vi "AutoRun.vi"(11 "AllControls In":T2) -> ()   [LabVIEW 2017]
uses:
  Ctrls/AllControls.ctl
  Ctrls/CSV_Data.ctl
  Ctrls/NFC.bat
  <vilib>/Utility/miscctls.llb/LVRowAndColumnTypeDef.ctl
  Ctrls/PathChoose.ctl
  ComVIS/Files/Ini/WriteIniFiles_ByVarient.vi
  <vilib>/Utility/file.llb/Write Delimited Spreadsheet (string).vi
  <vilib>/regexp/Match Regular Expression.xnode
panel:
  in  "Data in 2":T1
  in  "Data in":T1
types:
  T1 = typedef "CSV_Data.ctl" = cluster{"Version":cluster{"SC_Version":string, "VP_Version":string}, "SN":string, "Table":string[][], "Count":cluster{"Total":i32, "OK":i32, "NG":i32, "Yield":dbl}, "Start Time":timestamp, "daemon reference":refnum<k5>, "CT":dbl, "Config":string[][], "OK/NG":bool, "Station ID":string, "MES DDM SN":string, "MES PCBA SN":string, "Retest":string, "Lux":string, "VOT":cluster{"Initial brightness":string, "Mean uniformity":string, "Uniformity_Deviation":string, "Adjusted brightness":string, "Mean_Adjusted":string, "Deviation_Adjusted":string, "Reflection":string, "Result":bool}, "SKU":string, "Plate_Diameter":string, "Alarm":string}
  T2 = typedef "AllControls.ctl" = cluster{"MainVI":refnum<vi>, "AlarmInfo":refnum<vi>, "Log":refnum<vi>, "Current CT":refnum<vi>, "ProductID":refnum<vi>, "Device state":refnum<vi>, "MES":refnum<vi>, "mode":refnum<vi>, "TestInfo":refnum<vi>, "SubPnl":refnum<vi>, "Table":refnum<vi>, "MES bool":refnum<vi>, "TestMode":refnum<vi>, "Recipe":refnum<vi>, "Fail resume":refnum<vi>, "LogIn":refnum<vi>, "Start":refnum<vi>, "Maintenance":refnum<vi>, "Stop":refnum<vi>, "Exit":refnum<vi>}
  T3 = typedef "NFC.bat" = cluster{"getVersion":string, "Start Test mode":string, "Start camera test mode":string, "get one RAW Image":string, "Stop camera test mode":string, "Stop Test Mode":string, "Get image reflection":string, "Get image uniformity andFlash LED brightness":string, "Disable flash LED":string, "Enable flash LED":string, "Software Reset":string, "Tune Flash LED brightness":string, "Start Camera calibration":string, "Verify OBC Setting":string}
  T4 = typedef "amc_Message Queue.ctl" = refnum<queue>
  T5 = typedef "TesterInfo.ctl" = cluster{"Station Name":string, "Station Code":string, "ES NO.":string, "Tester ID":string, "PassMark Revision":string, "Rig ID":string, "682_Tool_Repeat":string, "Project Name":string, "FFTesterPath":path, "Enable_User":bool, "Mode":enum16{"682"}, "Fail_resume_mode":bool}
  T6 = cluster{"Total":i32, "OK":i32, "NG":i32, "Yield":dbl}
  T7 = typedef "LVRowAndColumnTypeDef.ctl" = cluster{"Row":i32, "Column":i32}
  T8 = enum8{"Enabled", "Disabled", "Disabled and Grayed Out"}
  T9 = typedef "PathChoose.ctl" = enum16{"OperatorLog", "AutoRunLog", "AlmLog", "TestData", "AllTestData", "backup_nvm", "backup_before_flashing"}
  T10 = typedef "HD Config.ctl" = cluster{" PC":cluster{"PC Address":u8[], "PC Port":i32}, "FCO":cluster{"COM":refnum<visa-resource-name>, "Baudrate":u32}, "DC Power ":cluster{"COM":refnum<visa-resource-name>, "Baudrate":u32}, "PW3336":cluster{"COM":refnum<visa-resource-name>, "Baudrate":u32}, "Lefoo":cluster{"COM":refnum<visa-resource-name>, "Baudrate":u32}, "Tempt&Hum":cluster{"COM":refnum<visa-resource-name>, "Baudrate":u32}, "DIPC":cluster{"COM":refnum<visa-resource-name>}, "Daemon":cluster{"IP Address":string, "Port":u16, "Retry":u16}, "NFC_Cmd":cluster{"COM":refnum<visa-resource-name>, "Baudrate":u32}, "Fail_resume_mode":bool, "GRR":bool, "NFC _Serial":cluster{"COM":refnum<visa-resource-name>, "Baudrate":u32}}
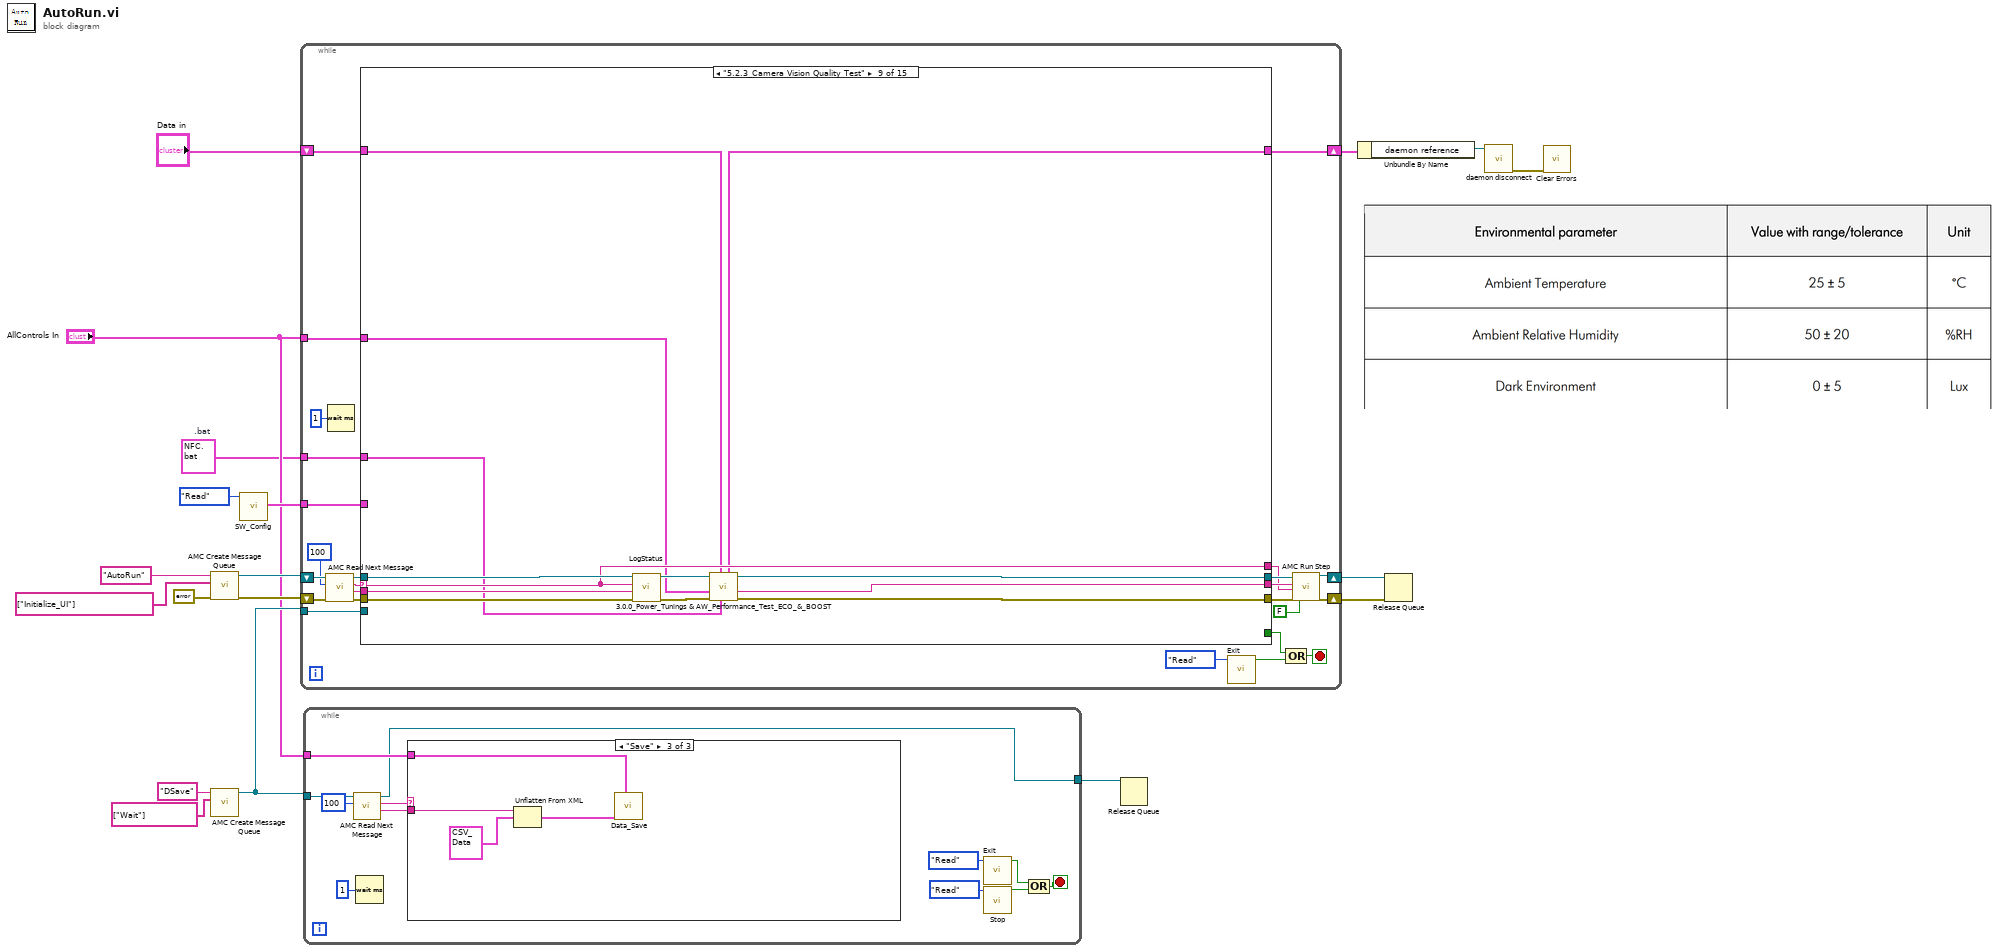
[diagram p0: block diagram]
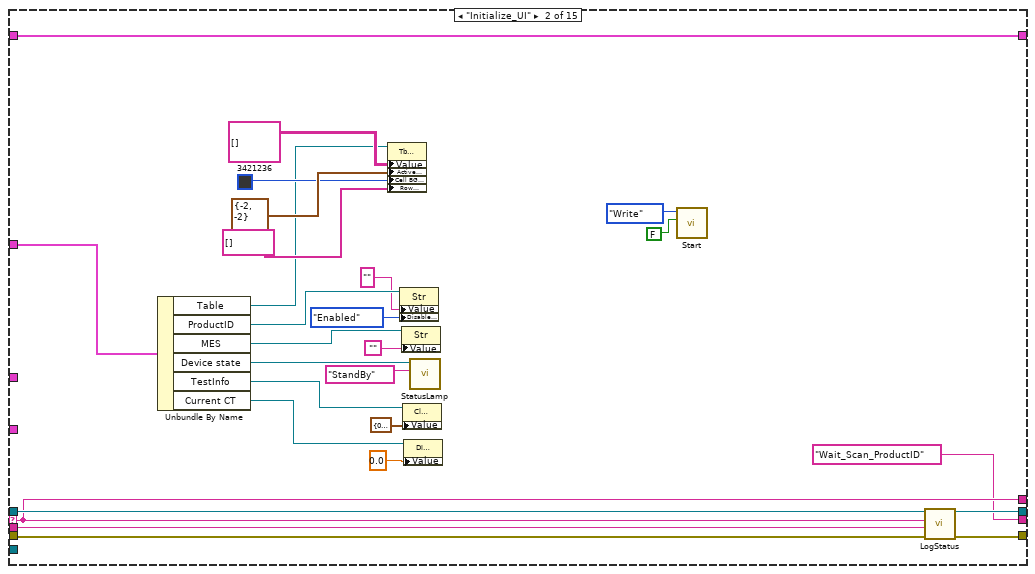
[diagram p5: hidden frame]
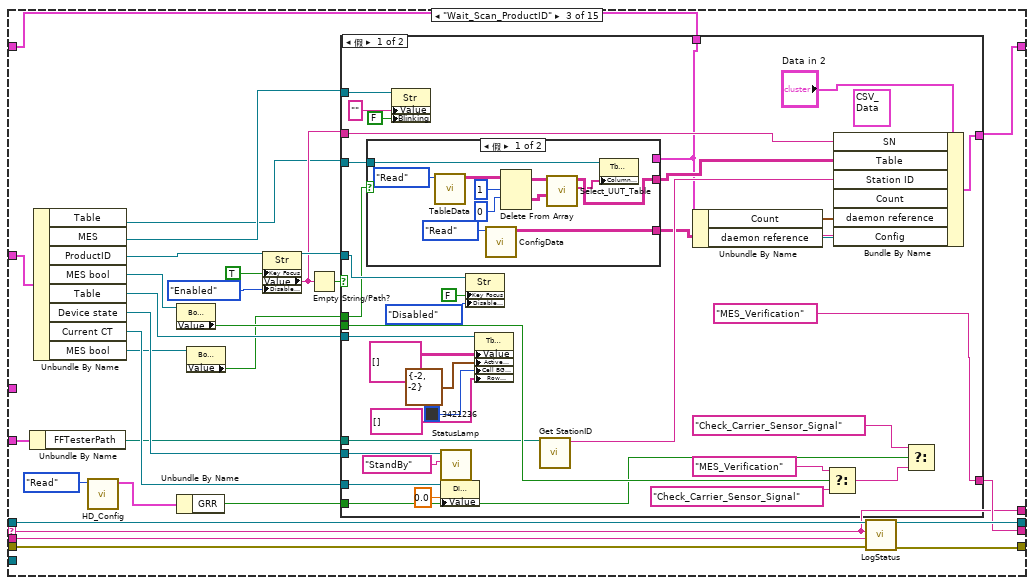
[diagram p6: hidden frame]
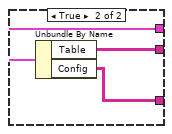
[diagram p7: hidden frame]
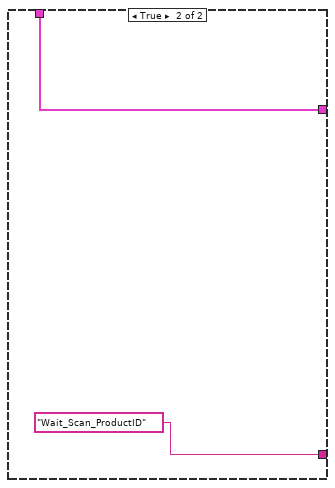
[diagram p8: hidden frame]
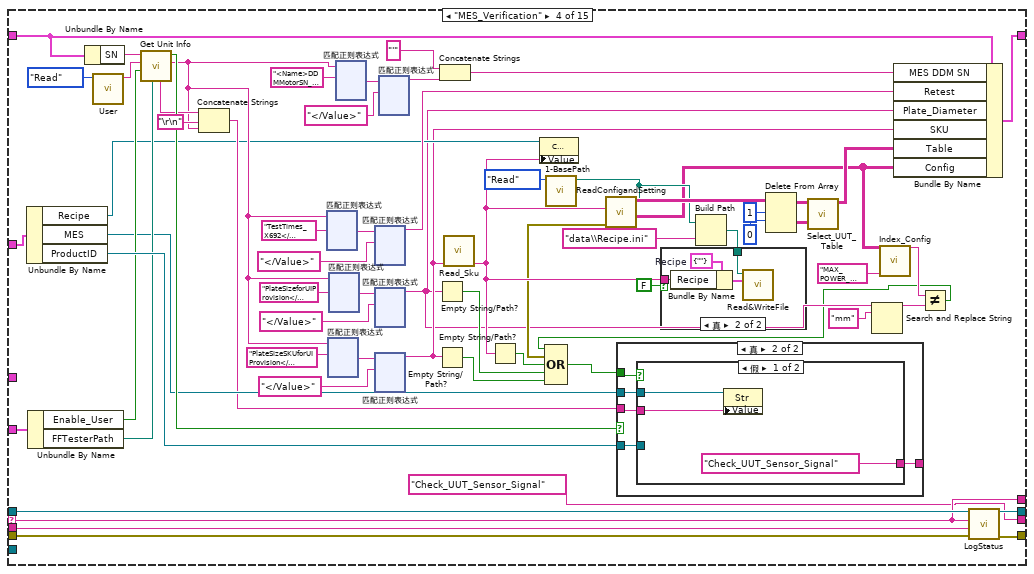
[diagram p9: hidden frame]
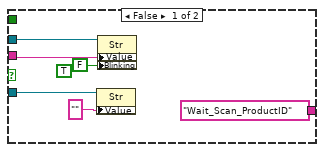
[diagram p11: hidden frame]
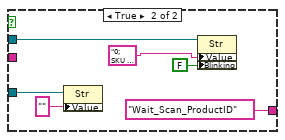
[diagram p12: hidden frame]
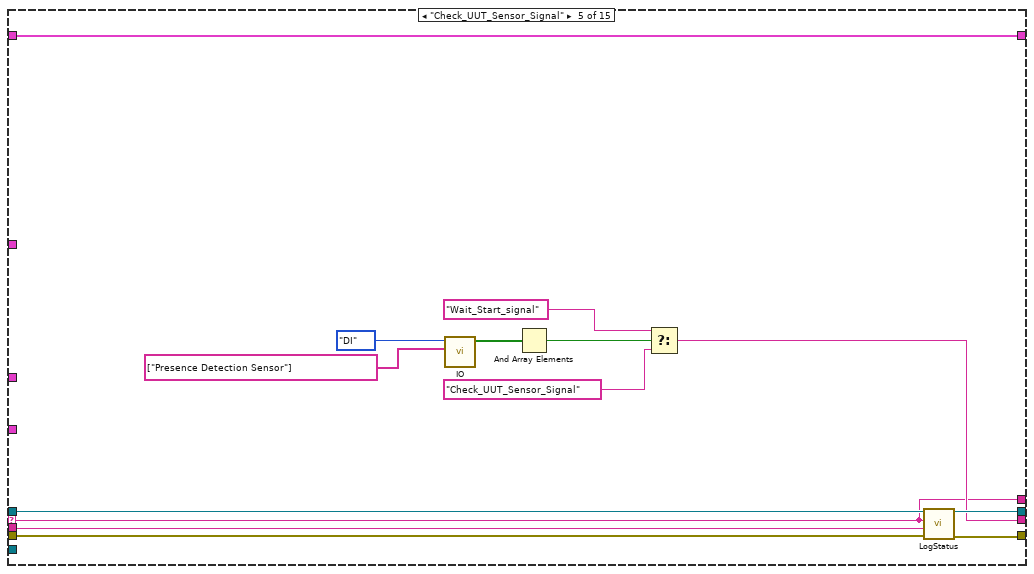
[diagram p13: hidden frame]
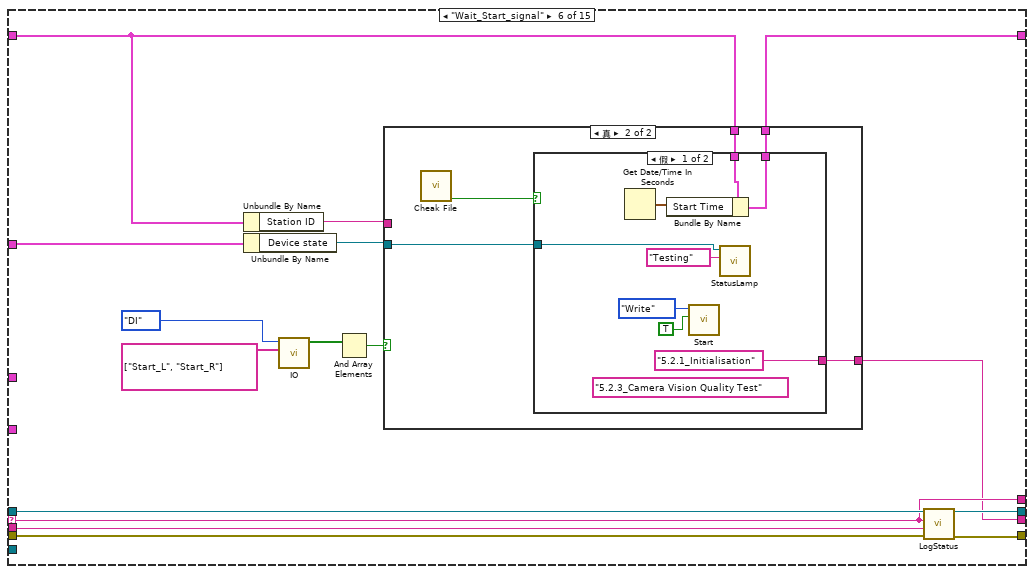
[diagram p14: hidden frame]
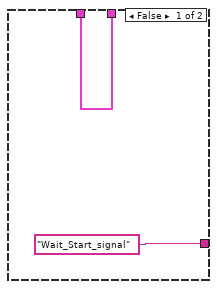
[diagram p15: hidden frame]
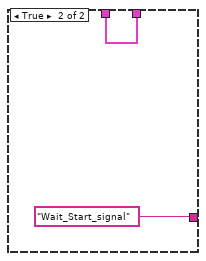
[diagram p16: hidden frame]
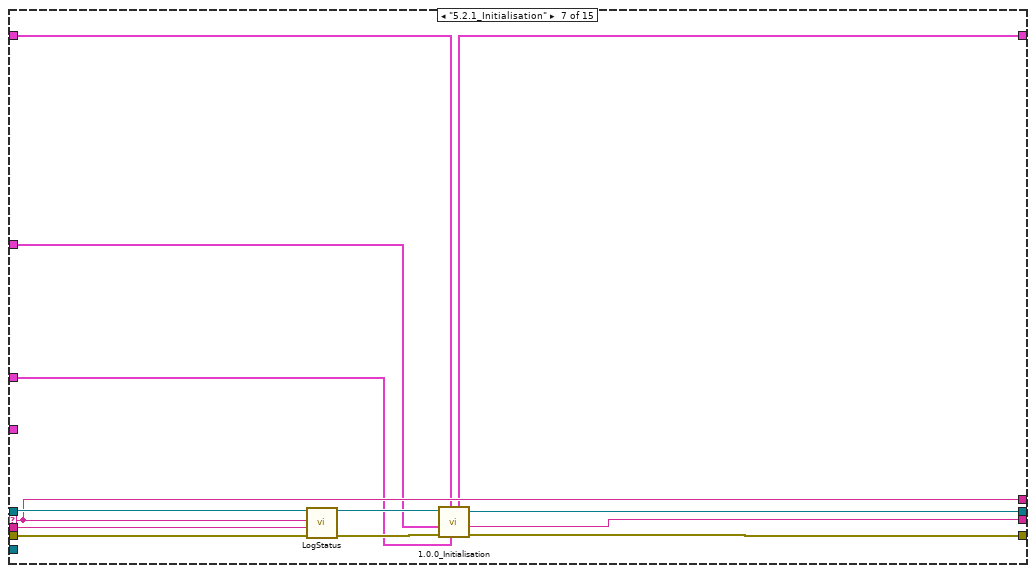
[diagram p17: hidden frame]
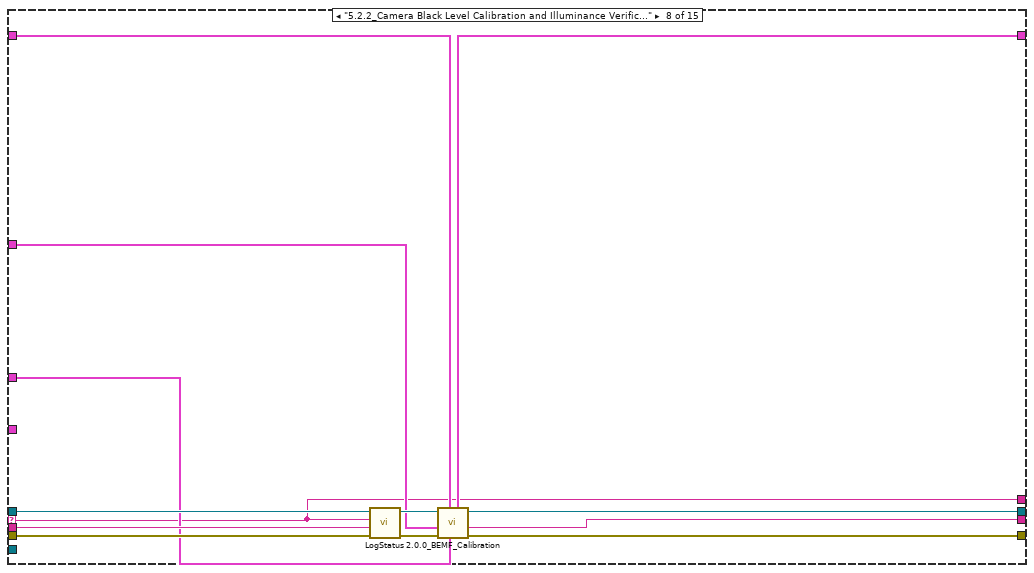
[diagram p18: hidden frame]
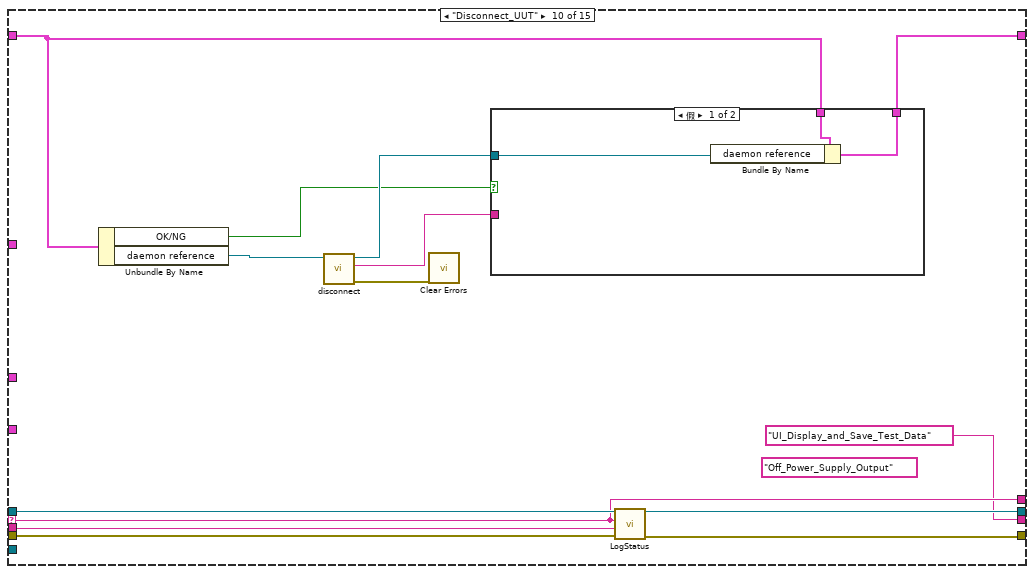
[diagram p19: hidden frame]
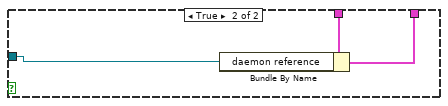
[diagram p20: hidden frame]
diagram:
  w1 = T3 {"getVersion"="Getting Software Version.bat", "Start Test mode"="Start Test Mode.bat", "Start camera test mode"="Start camera test mode.bat", "get one RAW Image"="Get one image.bat", "Stop camera test mode"="Stop camera test mode.bat", "Stop Test Mode"="Stop Test Mode.bat", "Get image reflection"="Get image reflection.bat", "Get image uniformity andFlash LED brightness"="Get image uniformity andFlash LED brightness.bat", "Disable flash LED"="Disable flash LED.bat", "Enable flash LED"="Enable flash LED.bat", "Software Reset"="Software Reset.bat", "Tune Flash LED brightness"="Tune Flash LED brightness.bat", "Start Camera calibration"="Start Camera calibration.bat", "Verify OBC Setting"="Verify OBC Setting.bat"}  # .bat
  n1 = call "AMC Create Message Queue.vi"("error in (no error)"=errorcluster {"status"=FALSE, "code"=0, "source"=""}, "Initial Message Names"=string[] ["Initialize_UI"] ("Initial Message Values"), "Message Queue Name"="AutoRun" ("Message queue name (unnamed)")) -> ("error out"=w17:errorcluster, "Message Queue out"=w18:T4)  [unwired: 2 in, 5 out]
  n2 = call "AMC Create Message Queue.vi"("Initial Message Names"=string[] ["Wait"], "Message Queue Name"="DSave") -> ("Message Queue out"=w13:T4)  [unwired: 3 in, 6 out]
  n3 = call "SW_Config.vi"("Step"=enum16{"Initial", "Write", "Read"}."Read") -> ("SW Config out"=w9:T5)  [unwired: 9 in, 1 out]
  n4 = while {
    tunnel: "AllControls In" -> [w30]
    shift-right: [w39] -> w6
    shift-left: w18 -> [w44]
    shift-right: [w40] -> w5
    shift-left: w17 -> [w43]
    tunnel: w13 -> [w35]
    tunnel: w9 -> [w23]
    shift-right: [w22] -> w8
    shift-left: "Data in" -> [w21]
    tunnel: w1 -> [w20]
    stop <- w38 stop-if-true
    n5 = call "AMC Read Next Message.vi"("error in (no error)"=w43, "timeout (1ms)"=100 ("Timeout"), "Message Queue in"=w44) -> ("error out"=w31:errorcluster, "Message Value"=w24:string, "Message Name"=w34:string, "Message Queue out"=w33:T4)  [unwired: 1 in, 4 out]
    n6 = Wait (ms)(milliseconds to wait=u32 1) -> ()  [unwired: 1 out]
    n7 = case shown="\"5.2.3_Camera Vision Quality Test\"" w34 {
      selector: w34 -> [_ w49 w90 w210 w1158 w1175 w1204 w1210 w1228 w1243 w1295 w1317 w1355 w1365 w1423]
      tunnel: w35 -> [_ _ _ _ _ _ _ _ _ _ w1299 _ _ _ _]
      tunnel: w33 -> [w47 w73 w102 w216 w1165 w1180 w1207 w1219 w1231 w1246 w1300 w1322 w1358 w1388 w1425]
      tunnel: [w47 w73 w102 w216 w1165 w1180 w1206 w1218 w1230 w1246 w1300 w1322 w1358 w1388 w1425] -> w32
      tunnel: w31 -> [w46 w53 w101 w215 w1164 w1179 w1209 w1221 w1233 w1245 w1297 w1321 w1357 w1387 w1421]
      tunnel: [w46 w69 w100 w214 w1163 w1178 w1205 w1217 w1229 w1244 w1296 w1320 w1356 w1386 w1422] -> w27
      tunnel: w30 -> [_ w71 w96 w212 _ w1171 w1202 w1214 w1225 _ w1286 w1302 w1346 w1376 _]
      tunnel: [_ _ _ _ _ _ _ _ _ _ _ _ _ _ TRUE] -> w29
      tunnel: [_ "Wait_Scan_ProductID" w94 "Check_UUT_Sensor_Signal" w1159 w1169 w1199 w1215 w1226 "UI_Display_and_Save_Test_Data" w1253 "Wait_Scan_ProductID" w1347 w1375 _] -> w26
      tunnel: [_ w49 w90 w210 w1158 w1175 w1204 w1210 w1228 w1243 w1295 w1317 w1355 w1365 _] -> w25
      tunnel: w24 -> [_ w63 w92 w211 w1157 w1174 w1208 w1220 w1232 w1242 w1294 w1318 w1354 w1364 _]
      tunnel: w23 -> [_ _ w83 w205 _ _ _ _ _ _ _ w1304 _ _ _]
      tunnel: [w45 w50 w81 w201 w1153 w1166 w1201 w1213 w1223 w1239 w1260 w1301 w1331 w1369 w1420] -> w22
      tunnel: w21 -> [w45 w50 w80 w202 w1153 w1167 w1200 w1212 w1224 w1238 w1259 w1301 w1331 w1370 w1420]
      tunnel: w20 -> [_ _ _ _ _ _ w1198 w1211 w1222 _ _ _ _ _ _]
      frame "Empty", Default {
      }
      frame "Initialize_UI" {
        n8 = Unbundle By Name(w71) -> ("Table"=w58:refnum<vi>, "ProductID"=w66:refnum<vi>, "MES"=w72:refnum<vi>, "Device state"=w68:refnum<vi>, "TestInfo"=w57:refnum<vi>, "Current CT"=w55:refnum<vi>)
        n9 = property class="Tbl (strict)"(reference=w58, "Value"=string[][] [] ("值"), "Active Cell"=T7 {"Row"=-2, "Column"=-2} ("活动单元格:活动单元格"), "Cell BG Color"=u32 3421236, "Row Headers[]"=string[] [] ("Row Header Strings[]")) -> ()  [unwired: 1 in, 2 out]
        n10 = property class="Str"(reference=w66, "Value"="" ("值"), "DisabledEnum"=T8."Enabled" ("Disabled")) -> ()  [unwired: 1 in, 2 out]
        n11 = property class="Str"(reference=w72, "Value"="") -> ()  [unwired: 1 in, 2 out]
        n12 = property class="Clust (strict)"(reference=w57, "Value"=T6 {"Total"=0, "OK"=0, "NG"=0, "Yield"=0.0}) -> ()  [unwired: 1 in, 2 out]
        n13 = property class="DigNum (strict)"(reference=w55, "Value"=0.0) -> ()  [unwired: 1 in, 2 out]
        n14 = call "StatusLamp.vi"("State"="StandBy", "Boolean输入"=w68) -> ()  [unwired: 9 in, 1 out]
        n15 = call "Start.vi"("Start In"=FALSE, "Step"=enum16{"Initial", "Write", "Read"}."Write") -> ()  [unwired: 8 in, 2 out]
        n16 = call "LogStatus.vi"("error in (no error)"=w53, "last message"=w63, "message"=w49) -> ("error  out"=w69:errorcluster)  [unwired: 8 in]
      }
      frame "Wait_Scan_ProductID" {
        n17 = Unbundle By Name(w83) -> ("FFTesterPath"=w82:path)
        n18 = Unbundle By Name(w96) -> ("Table"=w74:refnum<vi>, "MES"=w87:refnum<vi>, "ProductID"=w99:refnum<vi>, "MES bool"=w89:refnum<vi>, "Table"=w86:refnum<vi>, "Device state"=w85:refnum<vi>, "Current CT"=w84:refnum<vi>, "MES bool"=w76:refnum<vi>)
        n19 = call "HD_Config.vi"("Step"=enum16{"Initial", "Write", "Read"}."Read") -> ("HD Config out"=w78:T10)  [unwired: 9 in, 1 out]
        n20 = property class="Bool (strict)"(reference=w89) -> ("Value"=w88:bool)  [unwired: 1 in, 2 out]
        n21 = Unbundle By Name(w78) -> ("GRR"=w77:bool)
        n22 = property class="Bool (严格)"(reference=w76) -> ("Value"=w75:bool)  [unwired: 1 in, 2 out]
        n23 = property class="Str"(reference=w99, "Key Focus"=TRUE, "DisabledEnum"=T8."Enabled" ("Disabled")) -> (reference out=w93:refnum<vi>, "Value"=w91:string)  [unwired: 1 in, 1 out]
        n24 = Empty String/Path?(string/path=w91) -> (empty?=w95:bool)
        n25 = case shown="假" w95 {
          tunnel: ["MES_Verification" "Wait_Scan_ProductID"] -> w94
          tunnel: w93 -> [w134 _]
          tunnel: w91 -> [w117 _]
          tunnel: w88 -> [w131 _]
          tunnel: w87 -> [w130 _]
          tunnel: w86 -> [w124 _]
          tunnel: w85 -> [w122 _]
          tunnel: w84 -> [w121 _]
          tunnel: w82 -> [w119 _]
          tunnel: [w118 w151] -> w81
          tunnel: w80 -> [w105 w151]
          tunnel: w77 -> [w113 _]
          tunnel: w75 -> [w108 _]
          tunnel: w74 -> [w106 _]
          frame False {
            (unwired) T1 {"Version"={"SC_Version"="", "VP_Version"=""}, "SN"="", "Table"=[], "Count"={"Total"=0, "OK"=0, "NG"=0, "Yield"=0.0}, "Start Time"=timestamp(0 s since 1904-01-01), "daemon reference"=refnum, "CT"=0.0, "Config"=[], "OK/NG"=FALSE, "Station ID"="", "MES DDM SN"="", "MES PCBA SN"="", "Retest"="", "Lux"="", "VOT"={"Initial brightness"="", "Mean uniformity"="", "Uniformity_Deviation"="", "Adjusted brightness"="", "Mean_Adjusted"="", "Deviation_Adjusted"="", "Reflection"="", "Result"=FALSE}, "SKU"="", "Plate_Diameter"="", "Alarm"=""} ("Data in")
            n26 = case shown="假" w108 {
              tunnel: [w141 w149] -> w116
              tunnel: [w139 w148] -> w107
              tunnel: w106 -> [w138 _]
              tunnel: w105 -> [_ w150]
              frame False {
                n27 = call "TableData.vi"("Step"=enum16{"Initial", "Write", "Read"}."Read") -> ("Tabledata Out"=w142:string[][])  [unwired: 9 in, 1 out]
                n28 = call "ConfigData.vi"("Step"=enum16{"Initial", "Write", "Read"}."Read") -> ("Tabledata Out"=w139:string[][])  [unwired: 9 in, 1 out]
                n29 = Delete From Array(array=w142, length=1 ("长度"), index (row)=0 ("索引 (行)")) -> (deleted portion=w143:string[][], array with subset deleted=w144:string[][])  [unwired: 1 in]
                n30 = call "Select_UUT_Table.vi"("all Title"=w143, "all Table"=w144) -> ("Title"=w137:string[], "Table"=w141:string[][])  [unwired: 8 in]
                n31 = property class="Tbl (strict)"(reference=w138, "Column Headers[]"=w137) -> ()  [unwired: 1 in, 2 out]
              }
              frame True {
                n32 = Unbundle By Name(w150) -> ("Table"=w149:string[][], "Config"=w148:string[][])
              }
            }
            n33 = property class="Str"(reference=w130, "Value"="" ("值"), "Blinking"=FALSE ("闪烁")) -> ()  [unwired: 1 in, 2 out]
            n34 = call "StatusLamp.vi"("State"="StandBy", "Boolean输入"=w122) -> ()  [unwired: 9 in, 1 out]
            n35 = property class="DigNum (strict)"(reference=w121, "Value"=0.0) -> ()  [unwired: 1 in, 2 out]
            n36 = property class="Str"(reference=w134, "Key Focus"=FALSE, "DisabledEnum"=T8."Disabled" ("Disabled")) -> ()  [unwired: 1 in, 2 out]
            n37 = property class="Tbl (strict)"(reference=w124, "Value"=string[][] [] ("值"), "Active Cell"=T7 {"Row"=-2, "Column"=-2} ("活动单元格:活动单元格"), "Cell BG Color"=u32 3421236, "Row Headers[]"=string[] [] ("Row Header Strings[]")) -> ()  [unwired: 1 in, 2 out]
            n38 = call "Get StationID.vi"("路径"=w119) -> ("Station ID"=w115:string)  [unwired: 10 in]
            n39 = Unbundle By Name(w105) -> ("Count"=w111:T6, "daemon reference"=w110:refnum<k5>)
            n40 = Select(t="MES_Verification", s=w131, f="Check_Carrier_Sensor_Signal") -> (s? t:f=w114:string)
            n41 = Bundle By Name(cluster="Data in 2", "SN"=w117, "Table"=w116, "Station ID"=w115, "Count"=w111, "daemon reference"=w110, "Config"=w107) -> (w118:T1)
            n42 = Select(t="Check_Carrier_Sensor_Signal", s=w113, f=w114) -> ()  [unwired: 1 out]
          }
          frame True {
          }
        }
        n43 = call "LogStatus.vi"("error in (no error)"=w101, "last message"=w92, "message"=w90) -> ("error  out"=w100:errorcluster)  [unwired: 8 in]
      }
      frame "MES_Verification" {
        n44 = Unbundle By Name(w212) -> ("Recipe"=w167:refnum<vi>, "MES"=w188:refnum<vi>, "ProductID"=w208:refnum<vi>)
        n45 = Unbundle By Name(w205) -> ("Enable_User"=w204:bool, "FFTesterPath"=w203:path)
        n46 = Unbundle By Name(w202) -> ("SN"=w213:string)
        n47 = call "User.vi"("Step"=enum16{"Initial", "Write", "Read"}."Read") -> ("User out"=w206:string)  [unwired: 9 in, 1 out]
        n48 = call "Get Unit Info.vi"("路径"=w203, "Enable_User"=w204, "UserID"=w206, "Serial Number"=w213) -> ("strUnitInfo"=w180:string, "Operation Success"=w209:bool, "结果字符串"=w194:string)  [unwired: 2 in, 3 out]
        n49 = Concatenate Strings(w194, "\r\n", w180) -> (w187:string)
        n50 = xnode "匹配正则表达式"("输入字符串"=w180, "正则表达式"="TestTimes_X692</Name><Value>") -> ("匹配之后"=w192:string)  [unwired: 4 in, 4 out]
        n51 = xnode "匹配正则表达式"("输入字符串"=w180, "正则表达式"="PlateSizeSKUforUIProvision</Name><Value>") -> ("匹配之后"=w183:string)  [unwired: 4 in, 4 out]
        n52 = xnode "匹配正则表达式"("输入字符串"=w180, "正则表达式"="PlateSizeforUIProvision</Name><Value>") -> ("匹配之后"=w184:string)  [unwired: 4 in, 4 out]
        n53 = xnode "匹配正则表达式"("输入字符串"=w180, "正则表达式"="<Name>DDMMotorSN_X692</Name><Value>") -> ("匹配之后"=w198:string)  [unwired: 4 in, 4 out]
        n54 = xnode "匹配正则表达式"("输入字符串"=w192, "正则表达式"="</Value>") -> ("匹配之前"=w189:string)  [unwired: 4 in, 4 out]
        n55 = xnode "匹配正则表达式"("输入字符串"=w184, "正则表达式"="</Value>") -> ("匹配之前"=w156:string)  [unwired: 4 in, 4 out]
        n56 = xnode "匹配正则表达式"("输入字符串"=w183, "正则表达式"="</Value>") -> ("匹配之前"=w165:string)  [unwired: 4 in, 4 out]
        n57 = xnode "匹配正则表达式"("输入字符串"=w198, "正则表达式"="</Value>") -> ("匹配之前"=w197:string)  [unwired: 4 in, 4 out]
        n58 = Empty String/Path?(string/path=w156) -> (empty?=w179:bool)
        n59 = Empty String/Path?(string/path=w165) -> (empty?=w178:bool)
        n60 = Concatenate Strings("'", w197) -> (w196:string)
        n61 = call "Read_Sku.vi"("SKU"=w165) -> ("Recipe"=w164:string)  [unwired: 10 in]
        n62 = Empty String/Path?(string/path=w164) -> (empty?=w163:bool)
        n63 = property class="CmbBox"(reference=w167, "Value"=w164) -> ()  [unwired: 1 in, 2 out]
        n64 = call "1-BasePath.vi"("Step"=enum16{"Initial", "Write", "Read"}."Read") -> ("Path Out"=w173:path)  [unwired: 9 in, 1 out]
        n65 = call "ReadConfigandSetting.vi"("Recipe"=w164, "Path Out"=w173) -> ("错误输出"=w162:errorcluster, "ConfigData"=w157:string[][], "TableData"=w176:string[][])  [unwired: 7 in]
        n66 = Build Path(base path=w173, name or relative path="data\\Recipe.ini") -> (appended path=w172:path)
        n67 = case shown="真" FALSE {
          tunnel: w172 -> [_ w219]
          tunnel: w164 -> [_ w217]
          frame False {
          }
          frame True {
            w218 = cluster{"Recipe":string} {"Recipe"=""}  # Recipe
            n68 = Bundle By Name(cluster=w218, "Recipe"=w217) -> (w220:cluster{"Recipe":string})
            n69 = call-poly "Read&WriteFile.vi"("Variant"=w220, "path"=w219) -> ()  [unwired: 9 in, 1 out]
          }
        }
        n70 = Delete From Array(array=w176, length=1 ("长度"), index (row)=0 ("索引 (行)")) -> (deleted portion=w174:string[][], array with subset deleted=w175:string[][])  [unwired: 1 in]
        n71 = call "Select_UUT_Table.vi"("all Title"=w174, "all Table"=w175) -> ("Table"=w166:string[][])  [unwired: 8 in, 1 out]
        n72 = Search and Replace String(input string=w156, search string="mm" ("替换字符串(\"\")")) -> (result string=w160:string)  [unwired: 6 in, 3 out]
        n73 = call "Index_Config.vi"("Action"="MAX_POWER_MODE_Orifice_size", "config"=w157) -> ("data"=w159:string)  [unwired: 9 in]
        n74 = Bundle By Name(cluster=w202, "MES DDM SN"=w196, "Retest"=w189, "Plate_Diameter"=w156, "SKU"=w165, "Table"=w166, "Config"=w157) -> (w201:T1)
        n75 = Not Equal?(x=w159, y=w160) -> (x != y?=w155:bool)
        n76 = Compound Arithmetic op=OR ("复合运算")(w155, w162, w163, w179, w178) -> (w177:bool)
        n77 = case shown="真" w209 {
          tunnel: w208 -> [w1138 w1139]
          tunnel: ["Wait_Scan_ProductID" ("Value") w1143] -> _
          tunnel: w188 -> [w1135 w1142]
          tunnel: w187 -> [w1134 w1141]
          tunnel: w177 -> [_ w1140]
          frame False {
            (unwired) TRUE ("闪烁")
            n78 = property class="Str"(reference=w1138, "Value"="" ("值")) -> ()  [unwired: 1 in, 2 out]
            n79 = property class="Str"(reference=w1135, "Value"=w1134, "Blinking"=FALSE ("闪烁")) -> ()  [unwired: 1 in, 2 out]
          }
          frame True {
            n80 = case shown="假" w1140 {
              tunnel: ["Check_UUT_Sensor_Signal" "Wait_Scan_ProductID" ("Value")] -> w1143
              tunnel: w1142 -> [w1146 w1148]
              tunnel: w1141 -> [w1145 _]
              tunnel: w1139 -> [_ w1151]
              frame False {
                n81 = property class="Str"(reference=w1146, "Value"=w1145) -> ()  [unwired: 1 in, 2 out]
              }
              frame True {
                n82 = property class="Str"(reference=w1151, "Value"="" ("值")) -> ()  [unwired: 1 in, 2 out]
                n83 = property class="Str"(reference=w1148, "Value"="0; SKU or PlateSize Data Error" ("字符串"), "Blinking"=FALSE ("闪烁")) -> ()  [unwired: 1 in, 2 out]
              }
            }
          }
        }
        n84 = call "LogStatus.vi"("error in (no error)"=w215, "last message"=w211, "message"=w210) -> ("error  out"=w214:errorcluster)  [unwired: 8 in]
      }
      frame "Check_UUT_Sensor_Signal" {
        n85 = call "IO.vi"("IO Name"=string[] ["Presence Detection Sensor"], "IO?"=enum16{"DI", "DO"}."DI") -> ("DI"=w1156:bool[])  [unwired: 8 in, 1 out]
        n86 = And Array Elements(Boolean array=w1156) -> (logical AND=w1155:bool)
        n87 = Select(t="Wait_Start_signal", s=w1155, f="Check_UUT_Sensor_Signal") -> (s? t:f=w1159:string)
        n88 = call "LogStatus.vi"("error in (no error)"=w1164, "last message"=w1157, "message"=w1158) -> ("error  out"=w1163:errorcluster)  [unwired: 8 in]
      }
      frame "Wait_Start_signal" {
        n89 = Unbundle By Name(w1167) -> ("Station ID"=w1168:string)
        n90 = Unbundle By Name(w1171) -> ("Device state"=w1170:refnum<vi>)
        n91 = call "IO.vi"("IO Name"=string[] ["Start_L", "Start_R"], "IO?"=enum16{"DI", "DO"}."DI") -> ("DI"=w1173:bool[])  [unwired: 8 in, 1 out]
        n92 = And Array Elements(Boolean array=w1173) -> (logical AND=w1172:bool)
        n93 = case shown="真" w1172 {
          tunnel: w1170 -> [_ w1187]
          tunnel: w1167 -> [w1182 w1186]
          tunnel: [w1182 w1185] -> w1166
          tunnel: ["Wait_Start_signal" w1183] -> w1169
          tunnel: w1168 -> [_ _]
          frame False {
          }
          frame True {
            n94 = call "Cheak File.vi"() -> ("true"=w1184:bool)  [unwired: 11 in]
            n95 = case shown="假" w1184 {
              tunnel: w1187 -> [w1194 _]
              tunnel: w1186 -> [w1193 w1197]
              tunnel: [w1191 w1197] -> w1185
              tunnel: ["5.2.1_Initialisation" ("Name") "Wait_Start_signal"] -> w1183
              frame False {
                (unwired) "5.2.3_Camera Vision Quality Test"
                n96 = Get Date/Time In Seconds() -> (seconds since 1Jan1904=w1192:timestamp)
                n97 = Bundle By Name(cluster=w1193, "Start Time"=w1192) -> (w1191:T1)
                n98 = call "Start.vi"("Start In"=TRUE, "Step"=enum16{"Initial", "Write", "Read"}."Write") -> ()  [unwired: 8 in, 2 out]
                n99 = call "StatusLamp.vi"("State"="Testing", "Boolean输入"=w1194) -> ()  [unwired: 9 in, 1 out]
              }
              frame True {
              }
            }
          }
        }
        n100 = call "LogStatus.vi"("error in (no error)"=w1179, "last message"=w1174, "message"=w1175) -> ("error  out"=w1178:errorcluster)  [unwired: 8 in]
      }
      frame "5.2.1_Initialisation" {
        n101 = call "LogStatus.vi"("error in (no error)"=w1209, "last message"=w1208, "message"=w1204) -> ("error  out"=w1203:errorcluster)  [unwired: 8 in]
        n102 = call "1.0.0_Initialisation.vi"(".bat"=w1198, "Data in"=w1200, "error in (no error)"=w1203, "AllControls In"=w1202, "Message Queue out"=w1207) -> ("error out"=w1205:errorcluster, "Flow"=w1199:string, "Message Queue Out"=w1206:T4, "Data out"=w1201:T1)  [unwired: 3 in]
      }
      frame "5.2.2_Camera Black Level Calibration and Illuminance Verification" {
        n103 = call "LogStatus.vi"("error in (no error)"=w1221, "last message"=w1220, "message"=w1210) -> ("error  out"=w1216:errorcluster)  [unwired: 8 in]
        n104 = call "2.0.0_BEMF_Calibration.vi"(".bat"=w1211, "Data in"=w1212, "error in (no error)"=w1216, "AllControls In"=w1214, "Message Queue out"=w1219) -> ("error out"=w1217:errorcluster, "Flow"=w1215:string, "Message Queue Out"=w1218:T4, "Data out"=w1213:T1)  [unwired: 3 in]
      }
      frame "5.2.3_Camera Vision Quality Test" {
        n105 = call "LogStatus.vi"("error in (no error)"=w1233, "last message"=w1232, "message"=w1228) -> ("error  out"=w1227:errorcluster)  [unwired: 8 in]
        n106 = call "3.0.0_Power_Tunings & AW_Performance_Test_ECO_&_BOOST.vi"(".bat"=w1222, "Data in"=w1224, "error in (no error)"=w1227, "AllControls In"=w1225, "Message Queue out"=w1231) -> ("error out"=w1229:errorcluster, "Flow"=w1226:string, "Message Queue Out"=w1230:T4, "Data out"=w1223:T1)  [unwired: 3 in]
      }
      frame "Disconnect_UUT" {
        (unwired) "Off_Power_Supply_Output" ("Name")
        n107 = Unbundle By Name(w1238) -> ("OK/NG"=w1237:bool, "daemon reference"=w1240:refnum<k5>)
        n108 = call "disconnect.vi"("daemon reference in"=w1240) -> ("error out"=w1236:errorcluster, "response"=w1234:string, "daemon reference out"=w1241:refnum<k5>)  [unwired: 7 in, 1 out]
        n109 = call <vilib>:"Clear Errors.vi"("error in (no error)"=w1236) -> ()  [unwired: 5 in, 2 out]
        n110 = case shown="假" w1237 {
          tunnel: w1241 -> [w1247 w1252]
          tunnel: w1238 -> [w1248 w1251]
          tunnel: [w1249 w1250] -> w1239
          tunnel: w1234 -> [_ _]
          frame False {
            n111 = Bundle By Name(cluster=w1248, "daemon reference"=w1247) -> (w1249:T1)
          }
          frame True {
            n112 = Bundle By Name(cluster=w1251, "daemon reference"=w1252) -> (w1250:T1)
          }
        }
        n113 = call "LogStatus.vi"("error in (no error)"=w1245, "last message"=w1242, "message"=w1243) -> ("error  out"=w1244:errorcluster)  [unwired: 8 in]
      }
      frame "UI_Display_and_Save_Test_Data" {
        n114 = Unbundle By Name(w1286) -> ("ProductID"=w1272:refnum<vi>, "MES bool"=w1274:refnum<vi>, "Device state"=w1278:refnum<vi>, "TestInfo"=w1283:refnum<vi>, "Current CT"=w1285:refnum<vi>)
        n115 = Unbundle By Name(w1259) -> ("Start Time"=w1288:timestamp, "Count"=w1287:T6, "OK/NG"=w1269:bool)
        n116 = Get Date/Time In Seconds() -> (seconds since 1Jan1904=w1293:timestamp)
        n117 = Subtract(x=w1293, y=w1288) -> (x-y=w1279:dbl)
        n118 = property class="Str"(reference=w1272, "Value"="" ("值")) -> ()  [unwired: 1 in, 2 out]
        n119 = Unbundle By Name(w1287) -> ("Total"=w1292:i32, "OK"=w1266:i32, "NG"=w1267:i32)
        n120 = property class="DigNum (严格)"(reference=w1285, "Value"=w1279) -> ()  [unwired: 1 in, 2 out]
        n121 = Increment(x=w1292) -> (x+1=w1290:i32)
        n122 = Increment(x=w1266) -> (x+1=w1270:i32)
        n123 = Increment(x=w1267) -> (x+1=w1268:i32)
        n124 = Select(t=w1270, s=w1269, f=w1266) -> (s? t:f=w1265:i32)
        n125 = Select(t=w1267, s=w1269, f=w1268) -> (s? t:f=w1264:i32)
        n126 = Divide(x=w1265, y=w1290) -> (x/y=w1291:dbl)
        n127 = Multiply(x=w1291, y=100.0) -> (x*y=w1263:dbl)
        n128 = Bundle By Name(cluster=w1287, "Total"=w1290, "OK"=w1265, "NG"=w1264, "Yield"=w1263) -> (w1282:T6)
        n129 = Select(t="Pass" ("State"), s=w1269, f="Fail" ("State")) -> (s? t:f=w1277:string)
        n130 = call "StatusLamp.vi"("State"=w1277, "Boolean输入"=w1278) -> ()  [unwired: 9 in, 1 out]
        n131 = property class="Clust (严格)"(reference=w1283, "Value"=w1282) -> ()  [unwired: 1 in, 2 out]
        n132 = Bundle By Name(cluster=w1259, "CT"=w1279, "Count"=w1282) -> (w1260:T1)
        n133 = Flatten To XML(anything=w1260) -> (xml string=w1284:string)
        n134 = call "HD_Config.vi"("Step"=enum16{"Initial", "Write", "Read"}."Read") -> ("HD Config out"=w1257:T10)  [unwired: 9 in, 1 out]
        n135 = call "AMC Send Local Message.vi"("Message Value"=w1284, "Message Name"="Save", "Message Queue in"=w1299) -> ()  [unwired: 7 in, 2 out]
        n136 = property class="Bool (严格)"(reference=w1274) -> ("Value"=w1273:bool)  [unwired: 1 in, 2 out]
        n137 = Unbundle By Name(w1257) -> ("GRR"=w1256:bool)
        n138 = call "Start.vi"("Start In"=FALSE, "Step"=enum16{"Initial", "Write", "Read"}."Write") -> ()  [unwired: 8 in, 2 out]
        n139 = Select(t="Upload_MES_System", s=w1273, f="Wait_Scan_ProductID" ("Name")) -> (s? t:f=w1254:string)
        n140 = call "LogStatus.vi"("error in (no error)"=w1297, "last message"=w1294, "message"=w1295) -> ("error  out"=w1296:errorcluster)  [unwired: 8 in]
        n141 = Select(t="Wait_Scan_ProductID" ("Name"), s=w1256, f=w1254) -> (s? t:f=w1253:string)
      }
      frame "Upload_MES_System" {
        n142 = Unbundle By Name(w1304) -> ("Fail_resume_mode"=w1303:bool)
        n143 = Unbundle By Name(w1301) -> ("SN"=w1308:string, "OK/NG"=w1316:bool)
        n144 = Format Date/Time String(time format string (%c)="%H%M%S" ("时间格式字符串(%c)")) -> (date/time string=w1309:string)  [unwired: 2 in]
        n145 = call "PathChoose.vi"(11:PathChoose."TestData") -> ("Path_Out"=w1312:path)  [unwired: 10 in]
        n146 = Concatenate Strings(w1308, "_" ("字符串"), w1309, ".csv" ("字符串")) -> (w1306:string)
        n147 = call "Data_Table.vi"("AllControls In"=w1302, "Data in"=w1301) -> ("Data out"=w1315:string[][])  [unwired: 9 in]
        n148 = Build Path(base path=w1312, name or relative path=w1306) -> (appended path=w1311:path)
        n149 = call-poly <vilib>:"Write Delimited Spreadsheet.vi"("file path (dialog if empty)"=w1311, "2D data"=w1315, "delimiter (\\t)"="," ("delimiter (\\t)")) -> ()  [unwired: 11 in, 2 out]
        n150 = case shown="假" w1303 {
          tunnel: w1302 -> [w1330 _]
          tunnel: w1316 -> [w1326 _]
          tunnel: w1315 -> [w1325 _]
          tunnel: w1308 -> [w1324 _]
          frame False {
            n151 = call "Save Result.vi"("Data"=w1325, "布尔"=w1326, "ProductID"=w1324) -> ("结果字符串"=w1328:string)  [unwired: 5 in, 3 out]
            n152 = Unbundle By Name(w1330) -> ("MES"=w1329:refnum<vi>)
            n153 = Not Equal?(x=w1328, y="0") -> (x != y?=w1327:bool)
            n154 = property class="Str"(reference=w1329, "Value"=w1328, "Blinking"=w1327) -> ()  [unwired: 1 in, 2 out]
          }
          frame True {
          }
        }
        n155 = call "LogStatus.vi"("error in (no error)"=w1321, "last message"=w1318, "message"=w1317) -> ("error  out"=w1320:errorcluster)  [unwired: 8 in]
      }
      frame "Error" {
        n156 = Unbundle By Name(w1331) -> ("daemon reference"=w1340:refnum<k5>)
        n157 = Unbundle By Name(w1346) -> ("Device state"=w1333:refnum<vi>, "ProductID"=w1345:refnum<vi>)
        n158 = property class="Str"(reference=w1345) -> ("Value"=w1344:string)  [unwired: 1 in, 2 out]
        n159 = Not A Number/Path/Refnum?(number/path/refnum=w1340) -> (NaN/Path/Refnum?=w1339:bool)
        n160 = Empty String/Path?(string/path=w1344) -> (empty?=w1343:bool)
        n161 = Select(t="Off_Power_Supply_Output", s=w1339, f="Disconnect_UUT") -> (s? t:f=w1337:string)
        n162 = call "6-AlarmStatus.vi"("Step"=enum16{"Initial", "Write", "Read"}."Read") -> ("AlarmValue Out"=w1341:bool[])  [unwired: 9 in, 1 out]
        n163 = call "IO.vi"("IO Name"=string[] ["Reset"], "IO?"=enum16{"DI", "DO"}."DI") -> ("DI"=w1352:bool[])  [unwired: 8 in, 1 out]
        n164 = Or Array Elements(Boolean array=w1341) -> (logical OR=w1335:bool)
        n165 = And Array Elements(Boolean array=w1352) -> (logical AND=w1334:bool)
        n166 = Not(x=w1335) -> (.not. x?=w1332:bool)
        n167 = Select(t="Initialize_UI" ("Name"), s=w1343, f=w1337) -> (s? t:f=w1349:string)
        n168 = And(x=w1332, y=w1334) -> ()  [unwired: 1 out]
        n169 = Select(t=w1349, s=w1332, f="Error" ("Name")) -> (s? t:f=w1347:string)
        n170 = case shown="真" w1332 {
          tunnel: w1333 -> [_ w1359]
          frame False {
          }
          frame True {
            n171 = call "StatusLamp.vi"("State"="Testing", "Boolean输入"=w1359) -> ()  [unwired: 9 in, 1 out]
          }
        }
        n172 = call "LogStatus.vi"("error in (no error)"=w1357, "last message"=w1354, "message"=w1355) -> ("error  out"=w1356:errorcluster)  [unwired: 8 in]
      }
      frame "Stop_E-Stop" {
        n173 = while {
          shift-right: [w1394] -> w1366
          shift-left: w1364 -> [w1393]
          tunnel: w1365 -> [w1394]
          tunnel: [w1393] -> w1367
          stop <- FALSE continue-if-true
          n174 = Wait (ms)(milliseconds to wait=u32 1 ("等待时间（毫秒）")) -> ()  [unwired: 1 out]
        }
        n175 = Unbundle By Name(w1376) -> ("Device state"=w1371:refnum<vi>, "ProductID"=w1380:refnum<vi>)
        n176 = property class="Str"(reference=w1380) -> ("Value"=w1379:string)  [unwired: 1 in, 2 out]
        n177 = Not Equal?(x=w1366, y=w1367) -> (x != y?=w1363:bool)
        n178 = Empty String/Path?(string/path=w1379) -> (empty?=w1378:bool)
        n179 = call "6-AlarmStatus.vi"("Step"=enum16{"Initial", "Write", "Read"}."Read") -> ("AlarmValue Out"=w1368:bool[])  [unwired: 9 in, 1 out]
        n180 = case shown="真" w1363 {
          tunnel: w1370 -> [w1395 w1416]
          tunnel: [w1395 w1415] -> w1369
          tunnel: w1368 -> [_ w1400]
          frame False {
          }
          frame True {
            w1396 = 1 ("长度")
            n181 = call "3-AlarmConfig.vi"("Step"=enum16{"Initial", "Write", "Read"}."Read") -> ("AlarmConfig Out"=w1413:string[][])  [unwired: 9 in, 1 out]
            n182 = Index Array ("索引数组")(array=w1413, index (col)=1 ("索引 (列)")) -> (element=w1398:string[])  [unwired: 1 in]
            n183 = Search 1D Array(1D array=w1398, element="Test Error" ("元素")) -> (index of element=w1397:i32)  [unwired: 1 in]
            n184 = Delete From Array(array=w1398, length=w1396, index=w1397) -> (array with subset deleted=w1402:string[])  [unwired: 1 out]
            n185 = Delete From Array(array=w1400, length=w1396, index=w1397) -> (array with subset deleted=w1401:bool[])  [unwired: 1 out]
            n186 = for {
              tunnel: w1402 -> [w1418] mode=indexing
              tunnel: w1401 -> [w1417] mode=indexing
              tunnel: [w1418] -> w1408
              stop <- w1417 stop-if-true
            }
            n187 = call <vilib>:"Space Constant.vi"() -> ("String"=w1409:string)
            n188 = Search and Replace String(replace all?=TRUE ("replace all? (F)"), input string=w1408, search string=";", replace string=w1409) -> (result string=w1404:string)  [unwired: 4 in, 3 out]
            n189 = call <vilib>:"Space Constant.vi"() -> ("String"=w1407:string)
            n190 = Search and Replace String(replace all?=TRUE ("replace all? (F)"), input string=w1404, search string="-", replace string=w1407) -> (result string=w1403:string)  [unwired: 4 in, 3 out]
            n191 = Bundle By Name(cluster=w1416, "Alarm"=w1403) -> (w1415:T1)
          }
        }
        n192 = call "IO.vi"("IO Name"=string[] ["Reset"], "IO?"=enum16{"DI", "DO"}."DI") -> ("DI"=w1384:bool[])  [unwired: 8 in, 1 out]
        n193 = Or Array Elements(Boolean array=w1368) -> (logical OR=w1373:bool)
        n194 = And Array Elements(Boolean array=w1384) -> (logical AND=w1372:bool)
        n195 = Not(x=w1373) -> (.not. x?=w1362:bool)
        n196 = Select(t="Initialize_UI" ("Name"), s=w1378, f="Disconnect_UUT") -> (s? t:f=w1381:string)
        n197 = And(x=w1362, y=w1372) -> ()  [unwired: 1 out]
        n198 = Select(t=w1381, s=w1362, f="Stop_E-Stop" ("Name")) -> (s? t:f=w1375:string)
        n199 = case shown="真" w1362 {
          tunnel: w1371 -> [_ w1390]
          frame False {
          }
          frame True {
            n200 = call "StatusLamp.vi"("State"="Testing", "Boolean输入"=w1390) -> ()  [unwired: 9 in, 1 out]
          }
        }
        n201 = call "LogStatus.vi"("error in (no error)"=w1387, "last message"=w1364, "message"=w1365) -> ("error  out"=w1386:errorcluster)  [unwired: 8 in]
      }
      frame "Exit_AutoRun" {
        n202 = case shown="真" FALSE {
          frame False {
          }
          frame True {
            n203 = call "HD_Config.vi"("Step"=enum16{"Initial", "Write", "Read"}."Read") -> ("HD Config out"=w1436:T10)  [unwired: 9 in, 1 out]
            n204 = Unbundle By Name(w1436) -> ("DC Power.COM"=w1429:refnum<visa-resource-name>)
            n205 = call "EX_Set_V_A.vi"("current"="0", "voltage"="0", "VISA resource name"=w1429) -> ("VISA资源名称输出"=w1428:refnum<visa-resource-name>)  [unwired: 7 in, 1 out]
            n206 = call "EX_OUT_On_Off.vi"("Mode"=enum16{"ON", "OFF"}."OFF", "VISA resource name"=w1428) -> ("error out"=w1432:errorcluster)  [unwired: 8 in, 1 out]
            n207 = call "Time Delay6"("error in (no error)"=w1432) -> ("error out"=w1427:errorcluster)  [unwired: 10 in]
            n208 = call "IO.vi"("错误常量"=w1427, "DO DATA"=bool[] [FALSE, FALSE, FALSE, FALSE, FALSE] ("Writel_IO"), "IO Name"=string[] ["VE+", "GND", "COMM", "WAKE", "4V5"], "IO?"=enum16{"DI", "DO"}."DO") -> ("error out"=w1426:errorcluster)  [unwired: 6 in, 1 out]
            n209 = call "ini_Cylinder.vi"("error IO"=w1426) -> ("error out"=w1439:errorcluster)  [unwired: 10 in]
            n210 = call <vilib>:"Clear Errors.vi"("error in (no error)"=w1439) -> ()  [unwired: 5 in, 2 out]
          }
        }
        n211 = call "LogStatus.vi"("error in (no error)"=w1421, "message"=w1423) -> ("error  out"=w1422:errorcluster)  [unwired: 9 in]
      }
    }
    n212 = call "Exit.vi"("Step"=enum16{"Initial", "Write", "Read"}."Read" ("step")) -> ("Exit Out"=w37:bool)  [unwired: 9 in, 1 out]
    n213 = Compound Arithmetic op=OR(w29, w37) -> (w38:bool)
    n214 = call "AMC Run Step.vi"("Message Queue In"=w32, "Message Name"=w26, "Message Value"=w25, "error in (no error)"=w27, "Mli/Sig"=FALSE) -> ("Message Queue Out"=w39:T4, "error out"=w40:errorcluster)  [unwired: 13 in]
  }
  n215 = while {
    tunnel: w13 -> [w1446]
    tunnel: "AllControls In" -> [w1441]
    tunnel: [w1440] -> w4
    stop <- w1447 stop-if-true
    n216 = call "AMC Read Next Message.vi"("timeout (1ms)"=100, "Message Queue in"=w1446) -> ("Message Value"=w1442:string, "Message Name"=w1445:string, "Message Queue out"=w1440:T4)  [unwired: 2 in, 5 out]
    n217 = Wait (ms)(milliseconds to wait=u32 1) -> ()  [unwired: 1 out]
    n218 = case shown="\"Save\"" w1445 {
      tunnel: w1442 -> [_ _ w1455]
      tunnel: w1441 -> [_ _ w1454]
      frame "Null", Default {
      }
      frame "Wait" {
      }
      frame "Save" {
        n219 = Unflatten From XML(xml string=w1455, type=T1 {"Version"={"SC_Version"="", "VP_Version"=""}, "SN"="", "Table"=[], "Count"={"Total"=0, "OK"=0, "NG"=0, "Yield"=0.0}, "Start Time"=timestamp(0 s since 1904-01-01), "daemon reference"=refnum, "CT"=0.0, "Config"=[], "OK/NG"=FALSE, "Station ID"="", "MES DDM SN"="", "MES PCBA SN"="", "Retest"="", "Lux"="", "VOT"={"Initial brightness"="", "Mean uniformity"="", "Uniformity_Deviation"="", "Adjusted brightness"="", "Mean_Adjusted"="", "Deviation_Adjusted"="", "Reflection"="", "Result"=FALSE}, "SKU"="", "Plate_Diameter"="", "Alarm"=""} ("Data in")) -> (value=w1452:T1)  [unwired: 1 in, 1 out]
        n220 = call "Data_Save.vi"("AllControls In"=w1454, "Data in"=w1452) -> ()  [unwired: 10 in]
      }
    }
    n221 = call "Exit.vi"("Step"=enum16{"Initial", "Write", "Read"}."Read" ("step")) -> ("Exit Out"=w1449:bool)  [unwired: 9 in, 1 out]
    n222 = call "Stop.vi"("Step"=enum16{"Initial", "Write", "Read"}."Read") -> ("Stop Out"=w1448:bool)  [unwired: 9 in, 1 out]
    n223 = Compound Arithmetic op=OR(w1449, w1448) -> (w1447:bool)
  }
  n224 = Release Queue(queue=w4) -> ()  [unwired: 2 in, 3 out]
  n225 = Unbundle By Name(w8) -> ("daemon reference"=w12:refnum<k5>)
  n226 = Release Queue(queue=w6, error in (no error)=w5) -> ()  [unwired: 1 in, 3 out]
  n227 = call "daemon disconnect.vi"("daemon reference in"=w12) -> ("error out"=w11:errorcluster)  [unwired: 10 in]
  n228 = call <vilib>:"Clear Errors.vi"("error in (no error)"=w11) -> ()  [unwired: 5 in, 2 out]
